vi "Set Data Value.vi"(8 "error in (no error)":errorcluster, 9 "Data":variant, 11 "nameInterface in":refnum<class "nameInterface.lvclass">) -> (0 "error out":errorcluster, 3 "nameInterface out":refnum<class "nameInterface.lvclass">)   [LabVIEW 2017, in "nameInterface.lvlib" / "nameInterface.lvclass"]
uses:
  nameInterface.lvclass
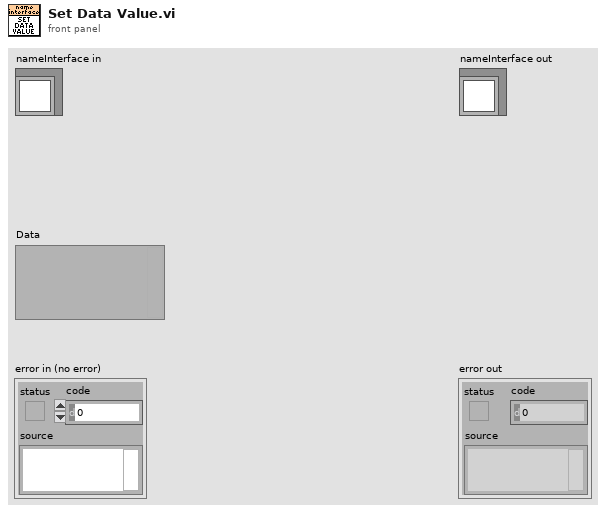
[diagram p1: front panel]
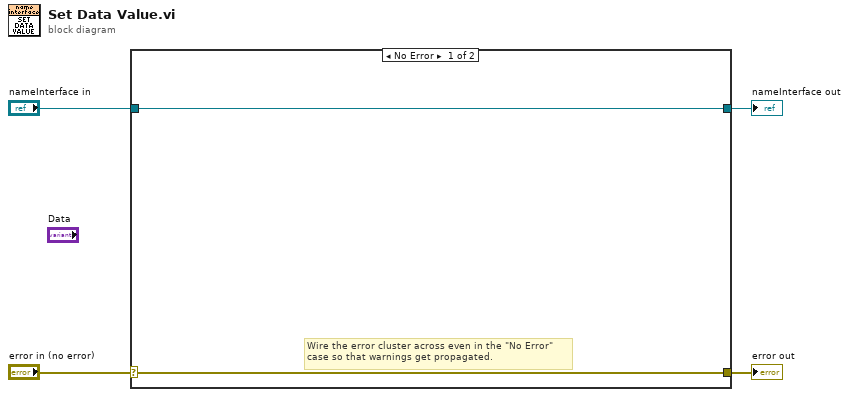
[diagram p0: block diagram]
diagram:
  n1 = case shown="No Error" "error in (no error)" {
    selector: "error in (no error)" -> [w5 w8]
    tunnel: [w5 w8] -> w3
    tunnel: [w6 w7] -> w1
    tunnel: "nameInterface in" -> [w6 w7]
    frame No Error {
      # "Wire the error cluster across even in the \"No Error\"\ncase so that warnings get propagated."
    }
    frame Error {
    }
  }
  "error out" <- w3
  "nameInterface out" <- w1
